vi "Data to Pedals Errors.vi"(1 "Data":u8[](array[numeric]) format="%b") -> (0 "Pedal Errors":T1)   [LabVIEW 2016]
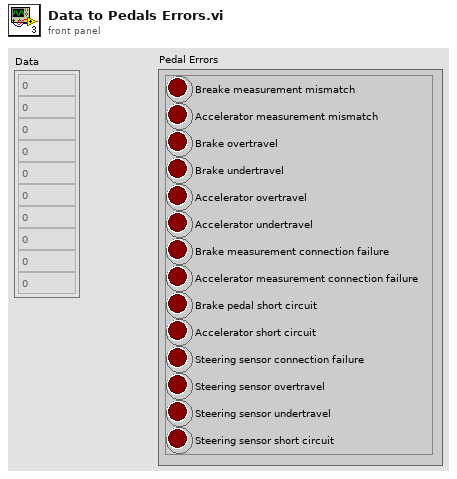
[diagram p1: front panel]
types:
  T1 = cluster{"Breake measurement mismatch":bool, "Accelerator overtravel":bool, "Brake pedal short circuit":bool, "Brake measurement connection failure":bool, "Steering sensor overtravel":bool, "Accelerator measurement connection failure":bool, "Brake undertravel":bool, "Steering sensor connection failure":bool, "Steering sensor short circuit":bool, "Steering sensor undertravel":bool, "Accelerator short circuit":bool, "Brake overtravel":bool, "Accelerator undertravel":bool, "Accelerator measurement mismatch":bool}
  T2 = cluster{"Boolean array[0]":bool, "Boolean array[1]":bool, "Boolean array[2]":bool, "Boolean array[3]":bool, "Boolean array[4]":bool, "Boolean array[5]":bool, "Boolean array[6]":bool, "Boolean array[7]":bool}
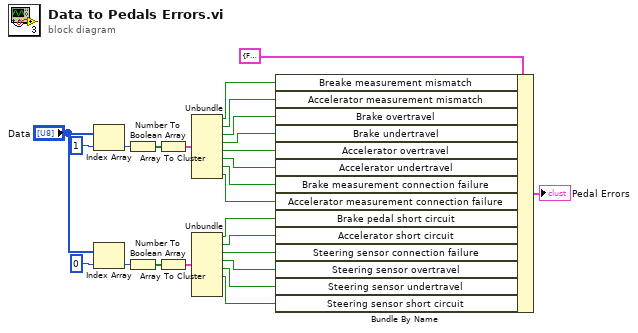
[diagram p0: block diagram]
diagram:
  n1 = Index Array(array="Data", index=1) -> (element=w22:u8)
  n2 = Index Array(array="Data", index=0) -> (element=w23:u8)
  n3 = Number To Boolean Array(number=w22) -> (Boolean array=w20:bool[])
  n4 = Number To Boolean Array(number=w23) -> (Boolean array=w21:bool[])
  n5 = Array To Cluster(array=w20) -> (cluster=w16:T2)
  n6 = Array To Cluster(array=w21) -> (cluster=w17:T2)
  n7 = Unbundle(w16) -> ("Boolean array[0]"=w15:bool, "Boolean array[1]"=w13:bool, "Boolean array[2]"=w12:bool, "Boolean array[3]"=w11:bool, "Boolean array[4]"=w10:bool, "Boolean array[5]"=w9:bool, "Boolean array[6]"=w8:bool, "Boolean array[7]"=w7:bool)
  n8 = Unbundle(w17) -> ("Boolean array[0]"=w6:bool, "Boolean array[1]"=w5:bool, "Boolean array[2]"=w4:bool, "Boolean array[3]"=w3:bool, "Boolean array[4]"=w2:bool, "Boolean array[5]"=w1:bool)  [unwired: 2 out]
  n9 = Bundle By Name(cluster=T1 {"Breake measurement mismatch"=FALSE, "Accelerator overtravel"=FALSE, "Brake pedal short circuit"=FALSE, "Brake measurement connection failure"=FALSE, "Steering sensor overtravel"=FALSE, "Accelerator measurement connection failure"=FALSE, "Brake undertravel"=FALSE, "Steering sensor connection failure"=FALSE, "Steering sensor short circuit"=FALSE, "Steering sensor undertravel"=FALSE, "Accelerator short circuit"=FALSE, "Brake overtravel"=FALSE, "Accelerator undertravel"=FALSE, "Accelerator measurement mismatch"=FALSE} ("Pedal Errors 2"), "Breake measurement mismatch"=w15, "Accelerator measurement mismatch"=w13, "Brake overtravel"=w12, "Brake undertravel"=w11, "Accelerator overtravel"=w10, "Accelerator undertravel"=w9, "Brake measurement connection failure"=w8, "Accelerator measurement connection failure"=w7, "Brake pedal short circuit"=w6, "Accelerator short circuit"=w5, "Steering sensor connection failure"=w4, "Steering sensor overtravel"=w3, "Steering sensor undertravel"=w2, "Steering sensor short circuit"=w1) -> (→"Pedal Errors":T1)
